vi "IECMemory.Stop.vi"(0 "i ref in":refnum<vi>, 3 "ms timeout (100)":i32=100, 5 "error in (no error)":errorcluster) -> (14 "i ref out":refnum<vi>, 17 "timed out":bool, 19 "error out":errorcluster)   [LabVIEW 2014, in "IECMemory.lvlib"]
uses:
  IECMemory.lvlib
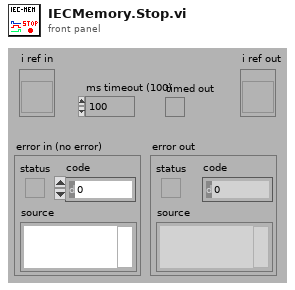
[diagram p1: front panel]
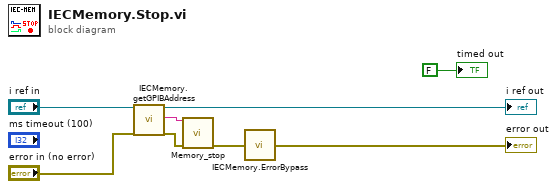
[diagram p0: block diagram]
diagram:
  n1 = call "IECMemory.getGPIBAddress.vi"("i ref in"="i ref in", "error in (no error)"="error in (no error)") -> ("i ref out"=→"i ref out":refnum<vi>, "GPIBAddress"=w5:string, "error out"=w6:errorcluster)  [unwired: 14 in, 1 out]
  n2 = call "Memory_stop.vi"("address string"=w5, "error in (no error)"=w6) -> ("error out"=w4:errorcluster)  [unwired: 12 in, 1 out]
  n3 = call "IECMemory.ErrorBypass.vi"("error in (no error)"=w4) -> ("error out"=→"error out":errorcluster)  [unwired: 14 in]
  "timed out" <- FALSE ("timed out")
